vi "re_install.vi"(8 "error in (no error)":errorcluster, 11 "post_installer-interface in":refnum<class "lv-post-installer.lvclass">) -> (0 "error out":errorcluster, 3 "post_installer-interface out":refnum<class "lv-post-installer.lvclass">)   [LabVIEW 2015, in "lv-post-installer.lvlib" / "lv-post-installer.lvclass"]
uses:
  lv-post-installer.lvclass
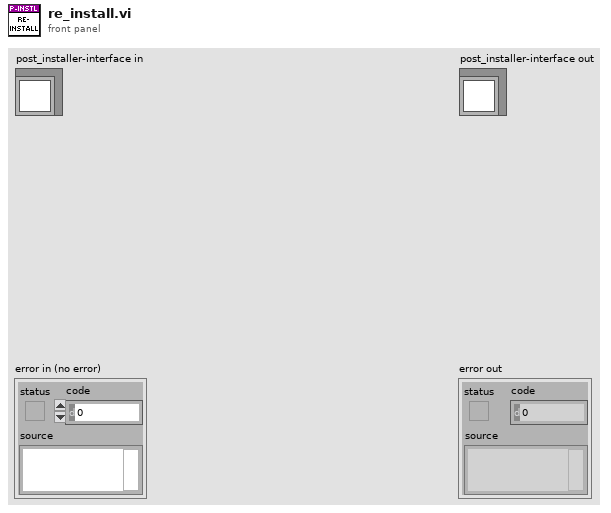
[diagram p1: front panel]
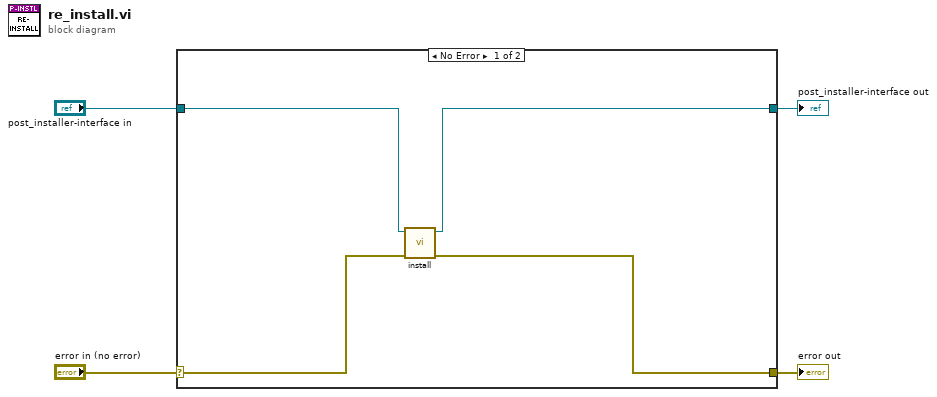
[diagram p0: block diagram]
diagram:
  n1 = case shown="No Error" "error in (no error)" {
    selector: "error in (no error)" -> [w6 w10]
    tunnel: [w5 w10] -> w3
    tunnel: [w7 w9] -> w1
    tunnel: "post_installer-interface in" -> [w8 w9]
    frame No Error {
      n2 = call-dynamic "install.vi"("error in (no error)"=w6, "plugin_interface in"=w8) -> ("error out"=w5:errorcluster, "plugin_interface out"=w7:refnum<class "lv-post-installer.lvclass">)  [unwired: 8 in]
    }
    frame Error {
    }
  }
  "error out" <- w3
  "post_installer-interface out" <- w1
